vi "PH_ImageCalibrator.ProcState.vi"(0 "i ref in":refnum<vi>, 2 "state timeout":i32=-1, 4 "state":string, 5 "error in (no error)":errorcluster) -> (14 "i ref out":refnum<vi>, 18 "next state":string, 19 "error out":errorcluster)   [LabVIEW 2014, in "PH_ImageCalibrator.lvlib"]
doc: "This VI represents part of the internal state machine of the object. All methods that are needed to implement the required functionality of the state machine will be called from THIS VI. Add your code here."
uses:
  PH_ImageCalibrator.lvlib
  CSCore/CSSystem/CoreDefs/CoreDefs.error_type.ctl
  CSCore/CSSystem/CoreLib/CoreLib.lvlib
  CSCore/BaseSM/BaseSM.lvlib
  CSCore/BaseProcess/BaseProcess.lvlib
  <vilib>/vision/NI_Vision_Development_Module.lvlib
  CSCore/CSSystem/CSSystemLib/CSSystemLib.lvlib
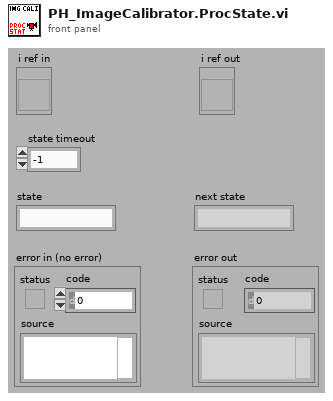
[diagram p1: front panel]
types:
  T1 = enum16{"simple", "synchronous", "asynchronous", "notification"}
  T2 = typedef "CoreDefs.error_type.ctl" = enum16{"no error", "can't load process", "can't unload process", "process does not exist", "can't install process", "can't remove process", "unknown function", "time out", "can't execute function", "duplicate queue name", "super not found", "caller queue invalid", "can't ping process", "unknown error", "VISA Error", "VISA timeout", "GPIB timeout", "GPIB error", "communication error", "data type mismatch", "can't read data from OPC server", "can't write data to OPC server", "OET error", "function not implemented", "process already exists", "invalid Shared Variable name", "error writing Shared Variable", "error reading Shared Variable", "invalid client name", "corrupt database", "unknown class", "call not authorized", "parameter out of range", "OET timeout: can't get data to modify", "invalid queue name", "requested operation incompatible with current state", "event undefined", "event disabled", "state undefined", "caller is not a friend", "EventBuilder: bad eventID", "EventBuilder: no DAQ devices", "a thread must not stop itself", "UNUSED ELEMENT4", "DiscArchiver: eventData incomplete", "DiscArchiver: eventData does not belong to run", "DiscArchiver: can't open file", "DiscArchiver: can't write to file", "DiscArchiver: available disc space low", "can't acquire semaphore", "error reading data from database", "notifier object is not existing", "can't register process", "can't unregister process", "illegal event type", "object disabled", "object already exists", "can't change state", "Instrument not found", "no connection to remote node", "invalid reference", "N/A", "UNUSED ELEMENT 1", "element not found", "illegal TCP/IP connection detected", "object does not exist", "invalid access ID", "unknown CS system", "invalid privilige", "unsupported data type", "unsupported server type", "IO server already exists", "Shared Variable already exists"}
  T3 = typedef "PH_ImageCalibrator.lvlib/PH_ImageCalibrator.i attribute.ctl" = cluster{"GUI Refs":cluster{"Available Cams":refnum<vi>, "OK":refnum<vi>, "Skip":refnum<vi>, "Repeat":refnum<vi>, "Cancel":refnum<vi>, "Length [mm]":refnum<vi>, "Energy [mJ]":refnum<vi>, "Dialog":refnum<vi>}, "Cam instances":string[], "Dark Pics":cluster{"#":i32, "BI taken":bool}, "Lin Cali":cluster{"Distance [Pixel]":dbl, "Distance [mm]":dbl, "Lin Cali Factor [mm/Pixel]":dbl}, "Energy Cali":cluster{"Pixelsum":dbl, "Energy [mJ]":dbl, "Energy Cali factor [mJ/Pixelsum]":dbl, "Underground subtracted?":bool, "#":i32}, "Images":cluster{"Background":T4, "Energy":T4}}
  T4 = typedef "IMAQ Image.ctl" = refnum<image>
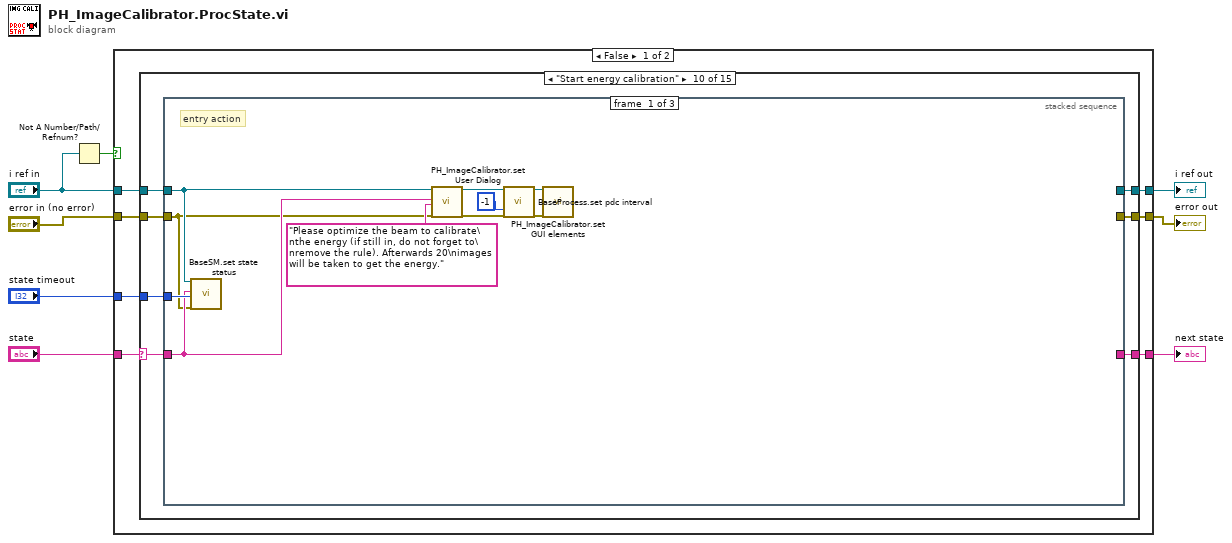
[diagram p0: block diagram]
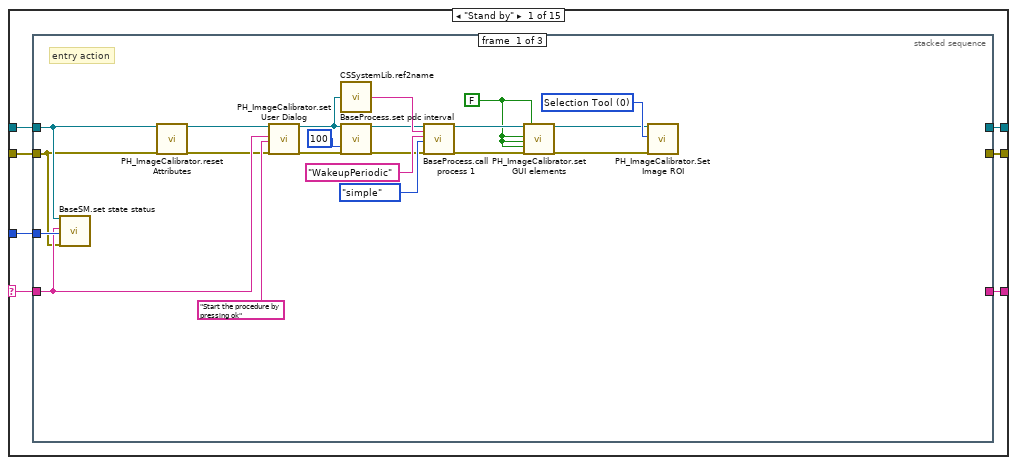
[diagram p2: hidden frame]
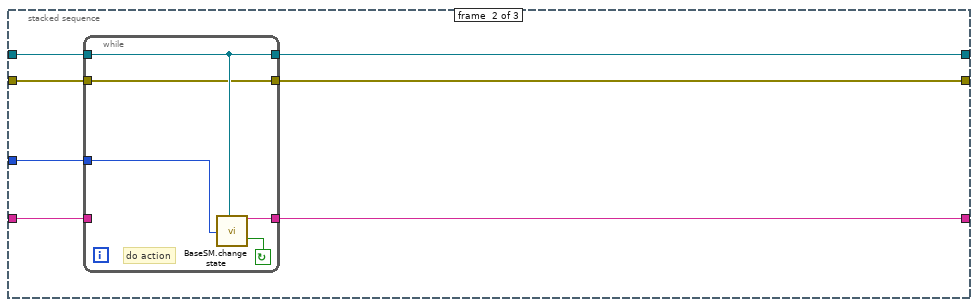
[diagram p3: hidden frame]
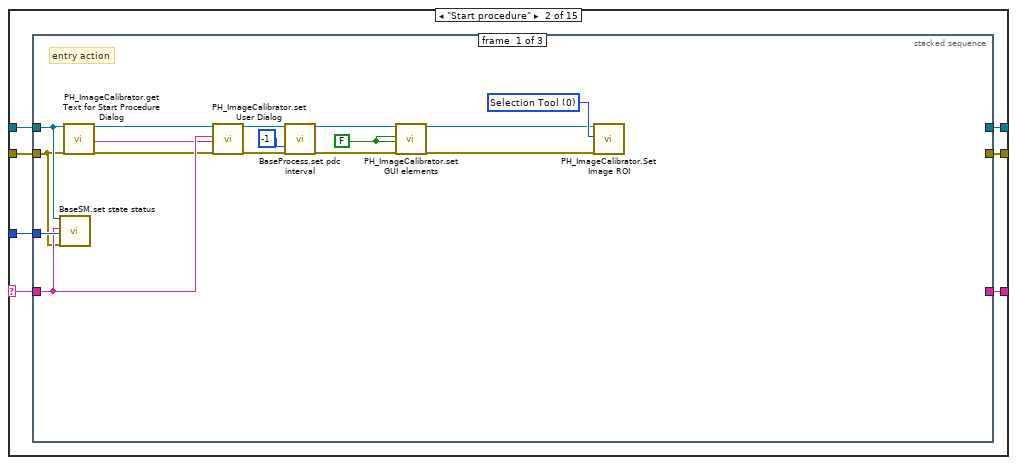
[diagram p5: hidden frame]
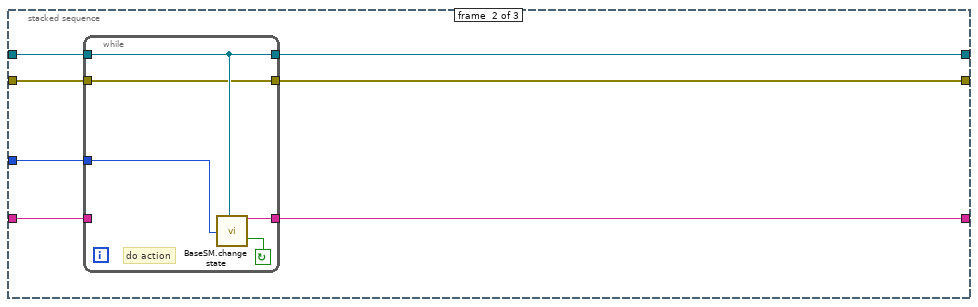
[diagram p6: hidden frame]
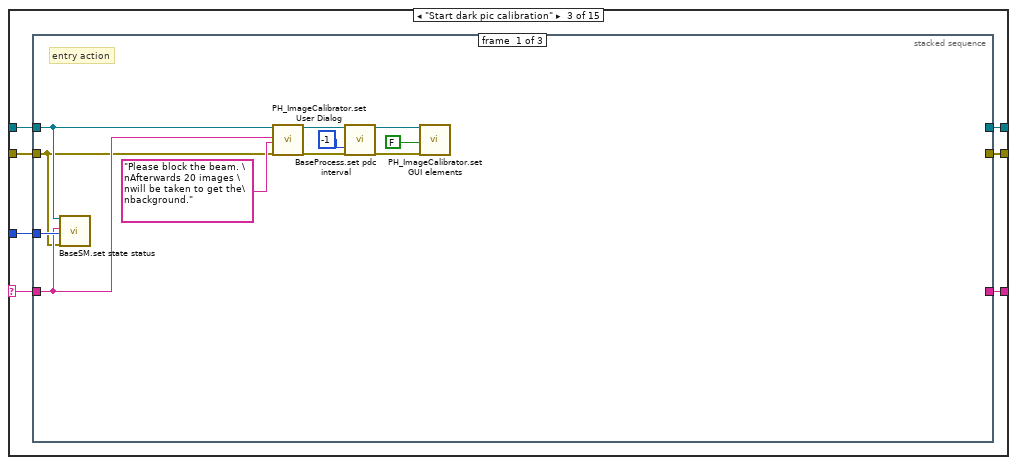
[diagram p8: hidden frame]
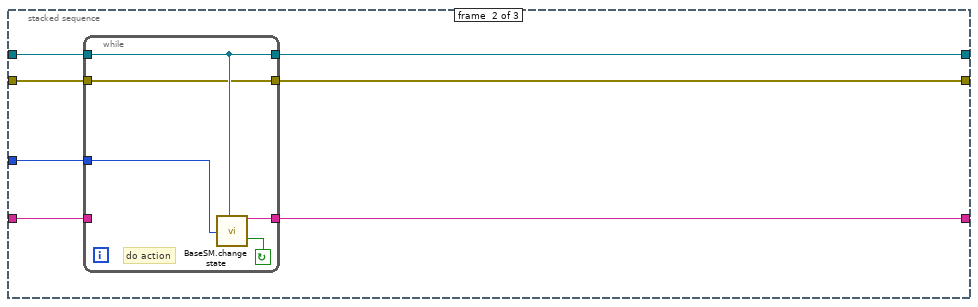
[diagram p9: hidden frame]
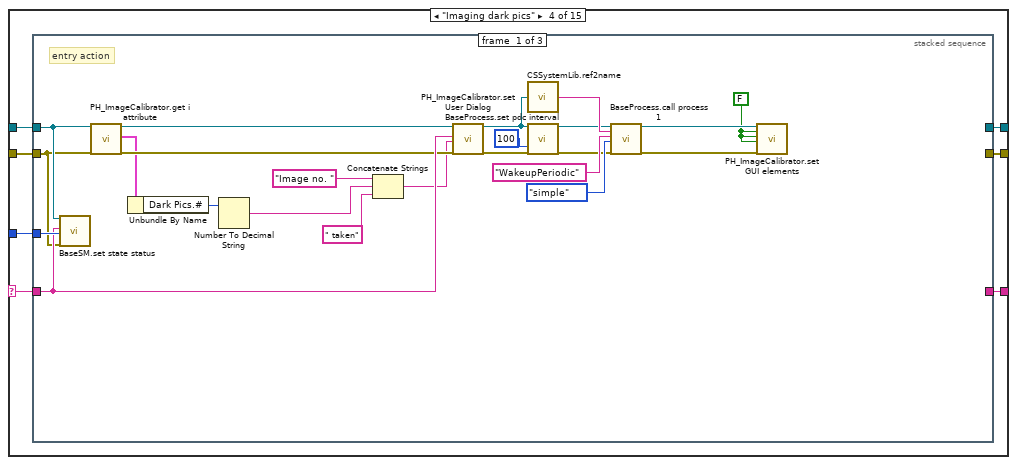
[diagram p11: hidden frame]
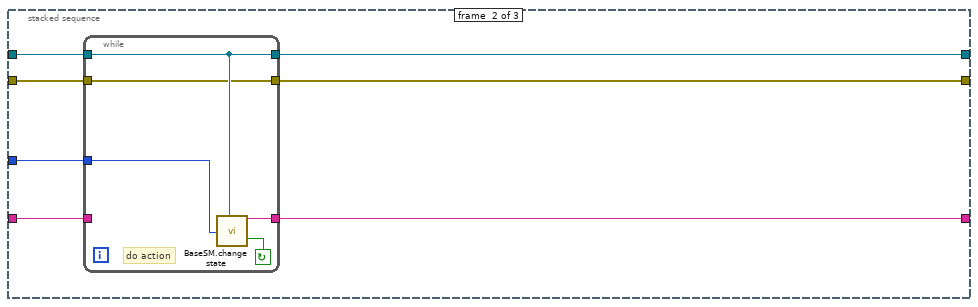
[diagram p12: hidden frame]
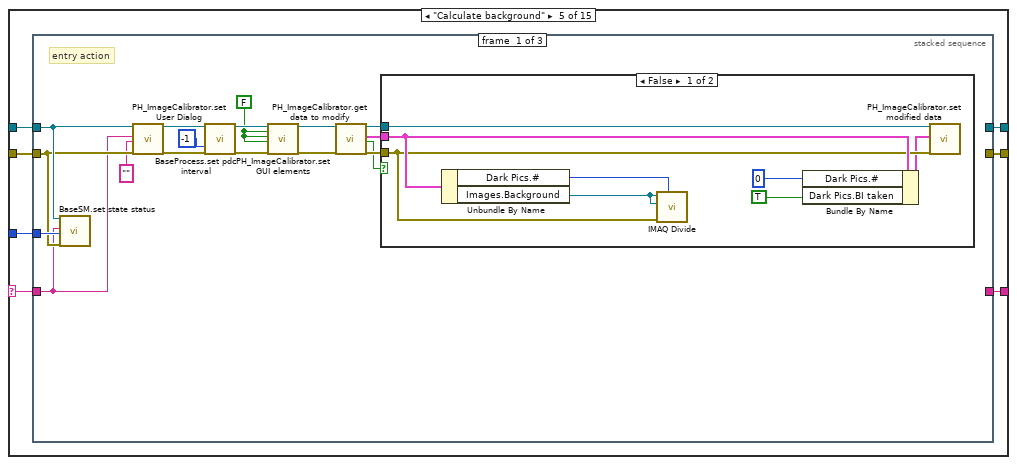
[diagram p14: hidden frame]
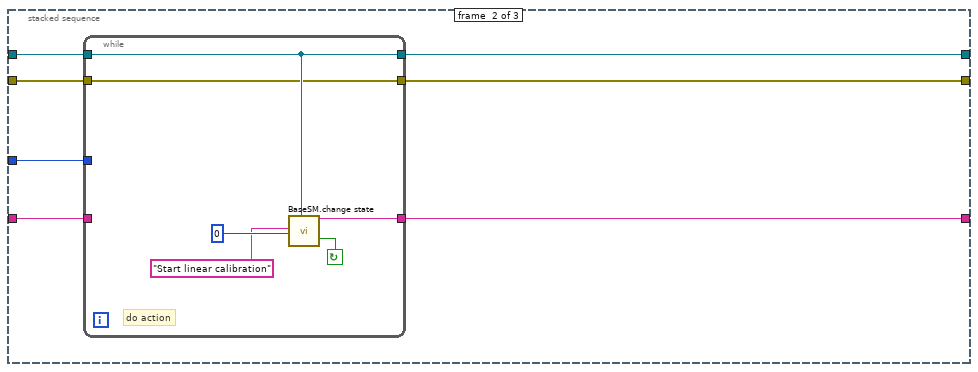
[diagram p16: hidden frame]
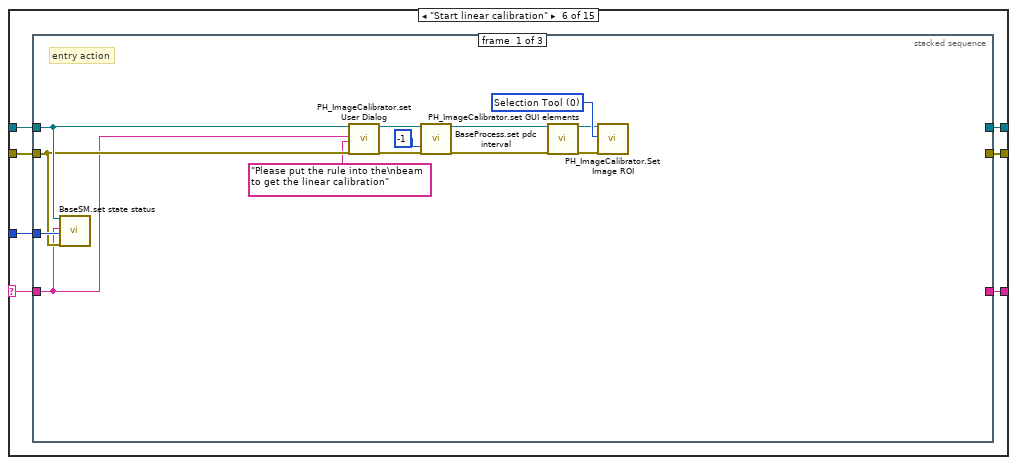
[diagram p18: hidden frame]
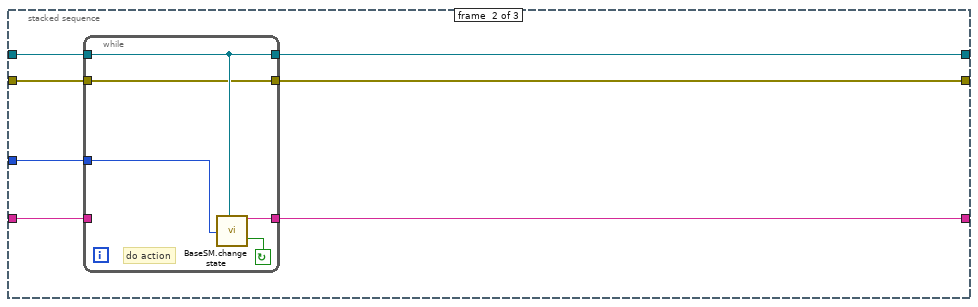
[diagram p19: hidden frame]
diagram:
  n1 = Not A Number/Path/Refnum?(number/path/refnum="i ref in") -> (NaN/Path/Refnum?=w2:bool)
  n2 = case shown="False" w2 {
    tunnel: "i ref in" -> [w15 w569]
    tunnel: [w14 w569] -> w8
    tunnel: "state" -> [w13 w566]
    tunnel: [w12 w566] -> w6
    tunnel: "state timeout" -> [w11 _]
    tunnel: "error in (no error)" -> [w10 _]
    tunnel: [w9 w567] -> w3
    frame False {
      n3 = case shown="\"Start energy calibration\"" w13 {
        selector: w13 -> [w22 w62 w97 w127 w169 w214 w246 w284 w316 w365 w394 w436 w484 w533 w560]
        tunnel: w15 -> [w20 w60 w95 w125 w167 w212 w244 w282 w314 w363 w392 w434 w482 w531 w565]
        tunnel: [w19 w59 w94 w124 w166 w211 w243 w281 w313 w362 w391 w433 w481 w530 w564] -> w14
        tunnel: [w21 w61 w96 w126 w168 w213 w245 w283 w315 w364 w393 w435 w483 w532 w559] -> w12
        tunnel: w11 -> [w18 w58 w93 w123 w165 w210 w242 w280 w312 w361 w390 w432 w480 w529 w561]
        tunnel: w10 -> [w17 w57 w92 w122 w164 w209 w241 w279 w311 w360 w389 w431 w479 w528 w563]
        tunnel: [w16 w56 w91 w121 w163 w208 w240 w278 w310 w359 w388 w430 w478 w527 w562] -> w9
        frame "Stand by" {
          n4 = stacked-sequence {
            tunnel: w22 -> [w42 w50 _]
            tunnel: [_ w49 _] -> w21
            tunnel: w20 -> [w29 w47 _]
            tunnel: [_ w46 _] -> w19
            tunnel: w18 -> [w43 w48 _]
            tunnel: w17 -> [w27 w44 _]
            tunnel: [_ w45 _] -> w16
            frame #0 {
              w25 = u32 0 items=["Zoom Tool"=8, "Selection Tool"=0, "Pan Tool"=9, "Point Tool"=1, "Line Tool"=2, "Rectangle Tool"=3, "Rotated Rectangle Tool"=12, "Polyline Tool"=10, "Polygon Tool"=5, "Freehand Tool"=11, "Closed Freehand Tool"=6, "Ellipse Tool"=4, "Annulus Tool"=7] ("ROI Tool")
              w30 = FALSE ("Cams disabled (true)")
              # "entry action"
              n5 = call "BaseSM.set state status.vi"("i ref in"=w29, "stateStatus"=w42, "ms timeout (10000)"=w43, "error in (no error)"=w27) -> ()  [unwired: 13 in, 3 out]
              n6 = call "PH_ImageCalibrator.reset Attributes.vi"("i ref in"=w29, "error in (no error)"=w27) -> ("i ref out"=w28:refnum<vi>, "error out"=w26:errorcluster)  [unwired: 16 in]
              n7 = call "PH_ImageCalibrator.set User Dialog.vi"("i ref in"=w28, "State"=w42, "Text"="Start the procedure by pressing ok", "error in (no error)"=w26) -> ("i ref out"=w34:refnum<vi>, "error out"=w36:errorcluster)  [unwired: 14 in]
              n8 = call "CSSystemLib.ref2name.vi"("obj refnum"=w34) -> ("name"=w40:string)
              n9 = call "BaseProcess.set pdc interval.vi"("i ref in"=w34, "PeriodicInterval [ms]"=100 ("PeriodicInterval"), "error in (no error)"=w36) -> ("i ref out"=w35:refnum<vi>, "error out"=w37:errorcluster)  [unwired: 14 in, 1 out]
              n10 = call "BaseProcess.call process 1.vi"("i ref in"=w35, "Object"=w40, "Selector"="WakeupPeriodic", "CallType"=T1."simple", "error in (no error)"=w37) -> ("i ref out"=w32:refnum<vi>, "error out"=w31:errorcluster)  [unwired: 12 in, 1 out]
              n11 = call "PH_ImageCalibrator.set GUI elements.vi"("i ref in"=w32, "skip visible (true)"=w30, "Repeat visible (true)"=w30, "Cancel visible (true)"=w30, "error in (no error)"=w31, "Cams disabled (true)"=w30) -> ("i ref out"=w24:refnum<vi>, "error out"=w23:errorcluster)  [unwired: 12 in]
              n12 = call "PH_ImageCalibrator.Set Image ROI.vi"("i ref in"=w24, "ROI Tool"=w25, "error in"=w23) -> ()  [unwired: 15 in, 2 out]
            }
            frame #1 {
              n13 = while {
                tunnel: w48 -> [w53]
                tunnel: [w55] -> w49
                tunnel: w50 -> [_]
                tunnel: w47 -> [w52]
                tunnel: [w52] -> w46
                tunnel: [w51] -> w45
                tunnel: w44 -> [w51]
                stop <- w54 continue-if-true
                # "do action"
                n14 = call "BaseSM.change state.vi"("wait time [ms]"=w53, "i ref in"=w52) -> ("next state"=w55:string, "continue loop"=w54:bool)  [unwired: 14 in, 2 out]
              }
            }
            frame #2 {
              # "exit action"
            }
          }
        }
        frame "Start procedure" {
          n15 = stacked-sequence {
            tunnel: w62 -> [w77 w85 _]
            tunnel: [_ w84 _] -> w61
            tunnel: w60 -> [w71 w82 _]
            tunnel: [_ w81 _] -> w59
            tunnel: w58 -> [w78 w83 _]
            tunnel: w57 -> [w69 w79 _]
            tunnel: [_ w80 _] -> w56
            frame #0 {
              w65 = u32 0 items=["Zoom Tool"=8, "Selection Tool"=0, "Pan Tool"=9, "Point Tool"=1, "Line Tool"=2, "Rectangle Tool"=3, "Rotated Rectangle Tool"=12, "Polyline Tool"=10, "Polygon Tool"=5, "Freehand Tool"=11, "Closed Freehand Tool"=6, "Ellipse Tool"=4, "Annulus Tool"=7] ("ROI Tool")
              w66 = FALSE ("Repeat visible (true)")
              # "entry action"
              n16 = call "BaseSM.set state status.vi"("i ref in"=w71, "stateStatus"=w77, "ms timeout (10000)"=w78, "error in (no error)"=w69) -> ()  [unwired: 13 in, 3 out]
              n17 = call "PH_ImageCalibrator.get Text for Start Procedure Dialog.vi"("i ref in"=w71, "error in (no error)"=w69) -> ("i ref out"=w70:refnum<vi>, "Dialog Start Procedure"=w67:string, "error out"=w68:errorcluster)  [unwired: 15 in]
              n18 = call "PH_ImageCalibrator.set User Dialog.vi"("i ref in"=w70, "State"=w77, "Text"=w67, "error in (no error)"=w68) -> ("i ref out"=w74:refnum<vi>, "error out"=w75:errorcluster)  [unwired: 14 in]
              n19 = call "BaseProcess.set pdc interval.vi"("i ref in"=w74, "PeriodicInterval [ms]"=-1 ("PeriodicInterval"), "error in (no error)"=w75) -> ("i ref out"=w73:refnum<vi>, "error out"=w72:errorcluster)  [unwired: 14 in, 1 out]
              n20 = call "PH_ImageCalibrator.set GUI elements.vi"("i ref in"=w73, "skip visible (true)"=w66, "Repeat visible (true)"=w66, "error in (no error)"=w72) -> ("i ref out"=w63:refnum<vi>, "error out"=w64:errorcluster)  [unwired: 14 in]
              n21 = call "PH_ImageCalibrator.Set Image ROI.vi"("i ref in"=w63, "ROI Tool"=w65, "error in"=w64) -> ()  [unwired: 15 in, 2 out]
            }
            frame #1 {
              n22 = while {
                tunnel: w83 -> [w88]
                tunnel: [w90] -> w84
                tunnel: w85 -> [_]
                tunnel: w82 -> [w87]
                tunnel: [w87] -> w81
                tunnel: [w86] -> w80
                tunnel: w79 -> [w86]
                stop <- w89 continue-if-true
                # "do action"
                n23 = call "BaseSM.change state.vi"("wait time [ms]"=w88, "i ref in"=w87) -> ("next state"=w90:string, "continue loop"=w89:bool)  [unwired: 14 in, 2 out]
              }
            }
            frame #2 {
              # "exit action"
            }
          }
        }
        frame "Start dark pic calibration" {
          n24 = stacked-sequence {
            tunnel: w97 -> [w107 w115 _]
            tunnel: [_ w114 _] -> w96
            tunnel: w95 -> [w99 w112 _]
            tunnel: [_ w111 _] -> w94
            tunnel: w93 -> [w108 w113 _]
            tunnel: w92 -> [w98 w109 _]
            tunnel: [_ w110 _] -> w91
            frame #0 {
              # "entry action"
              n25 = call "BaseSM.set state status.vi"("i ref in"=w99, "stateStatus"=w107, "ms timeout (10000)"=w108, "error in (no error)"=w98) -> ()  [unwired: 13 in, 3 out]
              n26 = call "PH_ImageCalibrator.set User Dialog.vi"("i ref in"=w99, "State"=w107, "Text"="Please block the beam. \nAfterwards 20 images \nwill be taken to get the\nbackground.", "error in (no error)"=w98) -> ("i ref out"=w104:refnum<vi>, "error out"=w105:errorcluster)  [unwired: 14 in]
              n27 = call "BaseProcess.set pdc interval.vi"("i ref in"=w104, "PeriodicInterval [ms]"=-1 ("PeriodicInterval"), "error in (no error)"=w105) -> ("i ref out"=w103:refnum<vi>, "error out"=w102:errorcluster)  [unwired: 14 in, 1 out]
              n28 = call "PH_ImageCalibrator.set GUI elements.vi"("i ref in"=w103, "Repeat visible (true)"=FALSE, "error in (no error)"=w102) -> ()  [unwired: 15 in, 2 out]
            }
            frame #1 {
              n29 = while {
                tunnel: w113 -> [w118]
                tunnel: [w120] -> w114
                tunnel: w115 -> [_]
                tunnel: w112 -> [w117]
                tunnel: [w117] -> w111
                tunnel: [w116] -> w110
                tunnel: w109 -> [w116]
                stop <- w119 continue-if-true
                # "do action"
                n30 = call "BaseSM.change state.vi"("wait time [ms]"=w118, "i ref in"=w117) -> ("next state"=w120:string, "continue loop"=w119:bool)  [unwired: 14 in, 2 out]
              }
            }
            frame #2 {
              # "exit action"
            }
          }
        }
        frame "Imaging dark pics" {
          n31 = stacked-sequence {
            tunnel: w127 -> [w149 w157 _]
            tunnel: [_ w156 _] -> w126
            tunnel: w125 -> [w148 w154 _]
            tunnel: [_ w153 _] -> w124
            tunnel: w123 -> [w150 w155 _]
            tunnel: w122 -> [w146 w151 _]
            tunnel: [_ w152 _] -> w121
            frame #0 {
              w128 = FALSE ("ok visible (true)")
              # "entry action"
              n32 = call "BaseSM.set state status.vi"("i ref in"=w148, "stateStatus"=w149, "ms timeout (10000)"=w150, "error in (no error)"=w146) -> ()  [unwired: 13 in, 3 out]
              n33 = call "PH_ImageCalibrator.get i attribute.vi"("i ref in"=w148, "error in (no error)"=w146) -> ("i ref out"=w147:refnum<vi>, "i attribute"=w144:T3, "error out"=w145:errorcluster)  [unwired: 15 in]
              n34 = Unbundle By Name(w144) -> ("Dark Pics.#"=w143:i32)
              n35 = Number To Decimal String(number=w143) -> (decimal integer string=w141:string)  [unwired: 1 in]
              n36 = Concatenate Strings("Image no. " ("string"), w141, " taken" ("string")) -> (w139:string)
              n37 = call "PH_ImageCalibrator.set User Dialog.vi"("i ref in"=w147, "State"=w149, "Text"=w139, "error in (no error)"=w145) -> ("i ref out"=w132:refnum<vi>, "error out"=w131:errorcluster)  [unwired: 14 in]
              n38 = call "CSSystemLib.ref2name.vi"("obj refnum"=w132) -> ("name"=w137:string)
              n39 = call "BaseProcess.set pdc interval.vi"("i ref in"=w132, "PeriodicInterval [ms]"=100 ("PeriodicInterval"), "error in (no error)"=w131) -> ("i ref out"=w133:refnum<vi>, "error out"=w134:errorcluster)  [unwired: 14 in, 1 out]
              n40 = call "BaseProcess.call process 1.vi"("i ref in"=w133, "Object"=w137, "Selector"="WakeupPeriodic", "CallType"=T1."simple", "error in (no error)"=w134) -> ("i ref out"=w130:refnum<vi>, "error out"=w129:errorcluster)  [unwired: 12 in, 1 out]
              n41 = call "PH_ImageCalibrator.set GUI elements.vi"("i ref in"=w130, "ok visible (true)"=w128, "skip visible (true)"=w128, "Repeat visible (true)"=w128, "error in (no error)"=w129) -> ()  [unwired: 13 in, 2 out]
            }
            frame #1 {
              n42 = while {
                tunnel: w155 -> [w160]
                tunnel: [w162] -> w156
                tunnel: w157 -> [_]
                tunnel: w154 -> [w159]
                tunnel: [w159] -> w153
                tunnel: [w158] -> w152
                tunnel: w151 -> [w158]
                stop <- w161 continue-if-true
                # "do action"
                n43 = call "BaseSM.change state.vi"("wait time [ms]"=w160, "i ref in"=w159) -> ("next state"=w162:string, "continue loop"=w161:bool)  [unwired: 14 in, 2 out]
              }
            }
            frame #2 {
              # "exit action"
            }
          }
        }
        frame "Calculate background" {
          n44 = stacked-sequence {
            tunnel: w169 -> [w183 w201 _]
            tunnel: [_ w200 _] -> w168
            tunnel: w167 -> [w185 w198 _]
            tunnel: [_ w197 _] -> w166
            tunnel: w165 -> [w186 w199 _]
            tunnel: w164 -> [w184 w195 _]
            tunnel: [_ w196 _] -> w163
            frame #0 {
              w176 = FALSE ("ok visible (true)")
              # "entry action"
              n45 = call "BaseSM.set state status.vi"("i ref in"=w185, "stateStatus"=w183, "ms timeout (10000)"=w186, "error in (no error)"=w184) -> ()  [unwired: 13 in, 3 out]
              n46 = call "PH_ImageCalibrator.set User Dialog.vi"("i ref in"=w185, "State"=w183, "Text"="", "error in (no error)"=w184) -> ("i ref out"=w180:refnum<vi>, "error out"=w181:errorcluster)  [unwired: 14 in]
              n47 = call "BaseProcess.set pdc interval.vi"("i ref in"=w180, "PeriodicInterval [ms]"=-1 ("PeriodicInterval"), "error in (no error)"=w181) -> ("i ref out"=w179:refnum<vi>, "error out"=w178:errorcluster)  [unwired: 14 in, 1 out]
              n48 = call "PH_ImageCalibrator.set GUI elements.vi"("i ref in"=w179, "ok visible (true)"=w176, "skip visible (true)"=w176, "Repeat visible (true)"=w176, "error in (no error)"=w178) -> ("i ref out"=w175:refnum<vi>, "error out"=w174:errorcluster)  [unwired: 13 in]
              n49 = call "PH_ImageCalibrator.get data to modify.vi"("i ref in"=w175, "error in (no error)"=w174) -> ("i ref out"=w170:refnum<vi>, "i attribute"=w173:T3, "timed out"=w171:bool, "error out"=w172:errorcluster)  [unwired: 14 in]
              n50 = case shown="False" w171 {
                tunnel: w173 -> [w193 _]
                tunnel: w172 -> [w191 _]
                tunnel: w170 -> [w192 _]
                frame False {
                  n51 = Unbundle By Name(w193) -> ("Dark Pics.#"=w194:i32, "Images.Background"=w187:T4)
                  n52 = call "IMAQ Divide"("Image Src A"=w187, "Constant"=w194, "Image Dst"=w187, "error in (no error)"=w191) -> ()  [unwired: 3 in, 2 out]
                  n53 = Bundle By Name(cluster=w193, "Dark Pics.#"=0, "Dark Pics.BI taken"=TRUE) -> (w190:T3)
                  n54 = call "PH_ImageCalibrator.set modified data.vi"("i ref in"=w192, "i attribute"=w190, "error in (no error)"=w191) -> ()  [unwired: 15 in, 2 out]
                }
                frame True {
                }
              }
            }
            frame #1 {
              n55 = while {
                tunnel: w199 -> [_]
                tunnel: [w207] -> w200
                tunnel: w201 -> [_]
                tunnel: w198 -> [w205]
                tunnel: [w205] -> w197
                tunnel: [w204] -> w196
                tunnel: w195 -> [w204]
                stop <- w206 continue-if-true
                # "do action"
                n56 = call "BaseSM.change state.vi"("default state"="Start linear calibration", "wait time [ms]"=0 ("wait time"), "i ref in"=w205) -> ("next state"=w207:string, "continue loop"=w206:bool)  [unwired: 13 in, 2 out]
              }
            }
            frame #2 {
              # "exit action"
            }
          }
        }
        frame "Start linear calibration" {
          n57 = stacked-sequence {
            tunnel: w214 -> [w224 w234 _]
            tunnel: [_ w233 _] -> w213
            tunnel: w212 -> [w226 w231 _]
            tunnel: [_ w230 _] -> w211
            tunnel: w210 -> [w227 w232 _]
            tunnel: w209 -> [w225 w228 _]
            tunnel: [_ w229 _] -> w208
            frame #0 {
              w217 = u32 0 items=["Zoom Tool"=8, "Selection Tool"=0, "Pan Tool"=9, "Point Tool"=1, "Line Tool"=2, "Rectangle Tool"=3, "Rotated Rectangle Tool"=12, "Polyline Tool"=10, "Polygon Tool"=5, "Freehand Tool"=11, "Closed Freehand Tool"=6, "Ellipse Tool"=4, "Annulus Tool"=7] ("ROI Tool")
              # "entry action"
              n58 = call "BaseSM.set state status.vi"("i ref in"=w226, "stateStatus"=w224, "ms timeout (10000)"=w227, "error in (no error)"=w225) -> ()  [unwired: 13 in, 3 out]
              n59 = call "PH_ImageCalibrator.set User Dialog.vi"("i ref in"=w226, "State"=w224, "Text"="Please put the rule into the\nbeam to get the linear calibration", "error in (no error)"=w225) -> ("i ref out"=w221:refnum<vi>, "error out"=w222:errorcluster)  [unwired: 14 in]
              n60 = call "BaseProcess.set pdc interval.vi"("i ref in"=w221, "PeriodicInterval [ms]"=-1 ("PeriodicInterval"), "error in (no error)"=w222) -> ("i ref out"=w220:refnum<vi>, "error out"=w219:errorcluster)  [unwired: 14 in, 1 out]
              n61 = call "PH_ImageCalibrator.set GUI elements.vi"("i ref in"=w220, "error in (no error)"=w219) -> ("i ref out"=w215:refnum<vi>, "error out"=w216:errorcluster)  [unwired: 16 in]
              n62 = call "PH_ImageCalibrator.Set Image ROI.vi"("i ref in"=w215, "ROI Tool"=w217, "error in"=w216) -> ()  [unwired: 15 in, 2 out]
            }
            frame #1 {
              n63 = while {
                tunnel: w232 -> [w237]
                tunnel: [w239] -> w233
                tunnel: w234 -> [_]
                tunnel: w231 -> [w236]
                tunnel: [w236] -> w230
                tunnel: [w235] -> w229
                tunnel: w228 -> [w235]
                stop <- w238 continue-if-true
                # "do action"
                n64 = call "BaseSM.change state.vi"("wait time [ms]"=w237, "i ref in"=w236) -> ("next state"=w239:string, "continue loop"=w238:bool)  [unwired: 14 in, 2 out]
              }
            }
            frame #2 {
              # "exit action"
            }
          }
        }
        frame "Imaging rule" {
          n65 = stacked-sequence {
            tunnel: w246 -> [w262 w272 _]
            tunnel: [_ w271 _] -> w245
            tunnel: w244 -> [w264 w269 _]
            tunnel: [_ w268 _] -> w243
            tunnel: w242 -> [w265 w270 _]
            tunnel: w241 -> [w263 w266 _]
            tunnel: [_ w267 _] -> w240
            frame #0 {
              w250 = u32 2 items=["Zoom Tool"=8, "Selection Tool"=0, "Pan Tool"=9, "Point Tool"=1, "Line Tool"=2, "Rectangle Tool"=3, "Rotated Rectangle Tool"=12, "Polyline Tool"=10, "Polygon Tool"=5, "Freehand Tool"=11, "Closed Freehand Tool"=6, "Ellipse Tool"=4, "Annulus Tool"=7] ("ROI Tool")
              # "entry action"
              n66 = call "BaseSM.set state status.vi"("i ref in"=w264, "stateStatus"=w262, "ms timeout (10000)"=w265, "error in (no error)"=w263) -> ()  [unwired: 13 in, 3 out]
              n67 = call "PH_ImageCalibrator.set User Dialog.vi"("i ref in"=w264, "State"=w262, "Text"="Please set a line as rule", "error in (no error)"=w263) -> ("i ref out"=w255:refnum<vi>, "error out"=w254:errorcluster)  [unwired: 14 in]
              n68 = call "CSSystemLib.ref2name.vi"("obj refnum"=w255) -> ("name"=w260:string)
              n69 = call "BaseProcess.set pdc interval.vi"("i ref in"=w255, "PeriodicInterval [ms]"=100 ("PeriodicInterval"), "error in (no error)"=w254) -> ("i ref out"=w256:refnum<vi>, "error out"=w257:errorcluster)  [unwired: 14 in, 1 out]
              n70 = call "BaseProcess.call process 1.vi"("i ref in"=w256, "Object"=w260, "Selector"="WakeupPeriodic", "CallType"=T1."simple", "error in (no error)"=w257) -> ("i ref out"=w253:refnum<vi>, "error out"=w252:errorcluster)  [unwired: 12 in, 1 out]
              n71 = call "PH_ImageCalibrator.set GUI elements.vi"("i ref in"=w253, "Repeat visible (true)"=FALSE, "error in (no error)"=w252) -> ("i ref out"=w248:refnum<vi>, "error out"=w249:errorcluster)  [unwired: 15 in]
              n72 = call "PH_ImageCalibrator.Set Image ROI.vi"("i ref in"=w248, "ROI Tool"=w250, "error in"=w249) -> ()  [unwired: 15 in, 2 out]
            }
            frame #1 {
              n73 = while {
                tunnel: w270 -> [w275]
                tunnel: [w277] -> w271
                tunnel: w272 -> [_]
                tunnel: w269 -> [w274]
                tunnel: [w274] -> w268
                tunnel: [w273] -> w267
                tunnel: w266 -> [w273]
                stop <- w276 continue-if-true
                # "do action"
                n74 = call "BaseSM.change state.vi"("wait time [ms]"=w275, "i ref in"=w274) -> ("next state"=w277:string, "continue loop"=w276:bool)  [unwired: 14 in, 2 out]
              }
            }
            frame #2 {
              # "exit action"
            }
          }
        }
        frame "Enter distance" {
          n75 = stacked-sequence {
            tunnel: w284 -> [w296 w304 _]
            tunnel: [_ w303 _] -> w283
            tunnel: w282 -> [w287 w301 _]
            tunnel: [_ w300 _] -> w281
            tunnel: w280 -> [w297 w302 _]
            tunnel: w279 -> [w288 w298 _]
            tunnel: [_ w299 _] -> w278
            frame #0 {
              w289 = FALSE ("Length not visible (true)")
              # "entry action"
              n76 = call "BaseSM.set state status.vi"("i ref in"=w287, "stateStatus"=w296, "ms timeout (10000)"=w297, "error in (no error)"=w288) -> ()  [unwired: 13 in, 3 out]
              n77 = call "PH_ImageCalibrator.set Distance in Pixel.vi"("i ref in"=w287, "error in (no error)"=w288) -> ("i ref out"=w286:refnum<vi>, "error out"=w285:errorcluster)  [unwired: 16 in]
              n78 = call "PH_ImageCalibrator.set User Dialog.vi"("i ref in"=w286, "State"=w296, "Text"="Please enter the length (in mm) for a nearfield cam,\nor the angle (in mrad) in case of a farfield cam,\nmarked within the auxiliary window", "error in (no error)"=w285) -> ("i ref out"=w293:refnum<vi>, "error out"=w294:errorcluster)  [unwired: 14 in]
              n79 = call "BaseProcess.set pdc interval.vi"("i ref in"=w293, "PeriodicInterval [ms]"=-1 ("PeriodicInterval"), "error in (no error)"=w294) -> ("i ref out"=w292:refnum<vi>, "error out"=w291:errorcluster)  [unwired: 14 in, 1 out]
              n80 = call "PH_ImageCalibrator.set GUI elements.vi"("i ref in"=w292, "ok visible (true)"=w289, "error in (no error)"=w291, "Length not visible (true)"=w289) -> ()  [unwired: 14 in, 2 out]
            }
            frame #1 {
              n81 = while {
                tunnel: w302 -> [w307]
                tunnel: [w309] -> w303
                tunnel: w304 -> [_]
                tunnel: w301 -> [w306]
                tunnel: [w306] -> w300
                tunnel: [w305] -> w299
                tunnel: w298 -> [w305]
                stop <- w308 continue-if-true
                # "do action"
                n82 = call "BaseSM.change state.vi"("wait time [ms]"=w307, "i ref in"=w306) -> ("next state"=w309:string, "continue loop"=w308:bool)  [unwired: 14 in, 2 out]
              }
            }
            frame #2 {
              # "exit action"
            }
          }
        }
        frame "Calculate linear calibration" {
          n83 = stacked-sequence {
            tunnel: w316 -> [w330 w352 _]
            tunnel: [_ w351 _] -> w315
            tunnel: w314 -> [w332 w349 _]
            tunnel: [_ w348 _] -> w313
            tunnel: w312 -> [w333 w350 _]
            tunnel: w311 -> [w331 w346 _]
            tunnel: [_ w347 _] -> w310
            frame #0 {
              w323 = FALSE ("ok visible (true)")
              # "entry action"
              n84 = call "BaseSM.set state status.vi"("i ref in"=w332, "stateStatus"=w330, "ms timeout (10000)"=w333, "error in (no error)"=w331) -> ()  [unwired: 13 in, 3 out]
              n85 = call "PH_ImageCalibrator.set User Dialog.vi"("i ref in"=w332, "State"=w330, "Text"="", "error in (no error)"=w331) -> ("i ref out"=w327:refnum<vi>, "error out"=w328:errorcluster)  [unwired: 14 in]
              n86 = call "BaseProcess.set pdc interval.vi"("i ref in"=w327, "PeriodicInterval [ms]"=-1 ("PeriodicInterval"), "error in (no error)"=w328) -> ("i ref out"=w326:refnum<vi>, "error out"=w325:errorcluster)  [unwired: 14 in, 1 out]
              n87 = call "PH_ImageCalibrator.set GUI elements.vi"("i ref in"=w326, "ok visible (true)"=w323, "skip visible (true)"=w323, "Repeat visible (true)"=w323, "error in (no error)"=w325) -> ("i ref out"=w318:refnum<vi>, "error out"=w317:errorcluster)  [unwired: 13 in]
              n88 = call "PH_ImageCalibrator.get data to modify.vi"("i ref in"=w318, "error in (no error)"=w317) -> ("i ref out"=w322:refnum<vi>, "i attribute"=w319:T3, "timed out"=w320:bool, "error out"=w321:errorcluster)  [unwired: 14 in]
              n89 = case shown="False" w320 {
                tunnel: w322 -> [w341 _]
                tunnel: w321 -> [w340 _]
                tunnel: w319 -> [w338 _]
                frame False {
                  n90 = Unbundle By Name(w338) -> ("Lin Cali.Distance [mm]"=w337:dbl, "Lin Cali.Distance [Pixel]"=w335:dbl)
                  n91 = Not Equal To 0?(x=w335) -> (x != 0?=w334:bool)
                  n92 = case shown="False" w334 {
                    tunnel: w337 -> [_ w345]
                    tunnel: w335 -> [_ w344]
                    tunnel: [1.0 w343] -> w336
                    frame False {
                    }
                    frame True {
                      n93 = Divide(x=w345, y=w344) -> (x/y=w343:dbl)
                    }
                  }
                  n94 = Bundle By Name(cluster=w338, "Lin Cali.Lin Cali Factor [mm/Pixel]"=w336) -> (w339:T3)
                  n95 = call "PH_ImageCalibrator.set modified data.vi"("i ref in"=w341, "i attribute"=w339, "error in (no error)"=w340) -> ()  [unwired: 15 in, 2 out]
                }
                frame True {
                }
              }
            }
            frame #1 {
              n96 = while {
                tunnel: w350 -> [_]
                tunnel: [w358] -> w351
                tunnel: w352 -> [_]
                tunnel: w349 -> [w356]
                tunnel: [w356] -> w348
                tunnel: [w355] -> w347
                tunnel: w346 -> [w355]
                stop <- w357 continue-if-true
                # "do action"
                n97 = call "BaseSM.change state.vi"("default state"="Start energy calibration", "wait time [ms]"=0 ("wait time"), "i ref in"=w356) -> ("next state"=w358:string, "continue loop"=w357:bool)  [unwired: 13 in, 2 out]
              }
            }
            frame #2 {
              # "exit action"
            }
          }
        }
        frame "Start energy calibration" {
          n98 = stacked-sequence {
            tunnel: w365 -> [w374 w382 _]
            tunnel: [_ w381 _] -> w364
            tunnel: w363 -> [w367 w379 _]
            tunnel: [_ w378 _] -> w362
            tunnel: w361 -> [w375 w380 _]
            tunnel: w360 -> [w366 w376 _]
            tunnel: [_ w377 _] -> w359
            frame #0 {
              # "entry action"
              n99 = call "BaseSM.set state status.vi"("i ref in"=w367, "stateStatus"=w374, "ms timeout (10000)"=w375, "error in (no error)"=w366) -> ()  [unwired: 13 in, 3 out]
              n100 = call "PH_ImageCalibrator.set User Dialog.vi"("i ref in"=w367, "State"=w374, "Text"="Please optimize the beam to calibrate\nthe energy (if still in, do not forget to\nremove the rule). Afterwards 20\nimages will be taken to get the energy.", "error in (no error)"=w366) -> ("i ref out"=w371:refnum<vi>, "error out"=w372:errorcluster)  [unwired: 14 in]
              n101 = call "BaseProcess.set pdc interval.vi"("i ref in"=w371, "PeriodicInterval [ms]"=-1 ("PeriodicInterval"), "error in (no error)"=w372) -> ("i ref out"=w370:refnum<vi>, "error out"=w369:errorcluster)  [unwired: 14 in, 1 out]
              n102 = call "PH_ImageCalibrator.set GUI elements.vi"("i ref in"=w370, "error in (no error)"=w369) -> ()  [unwired: 16 in, 2 out]
            }
            frame #1 {
              n103 = while {
                tunnel: w380 -> [w383]
                tunnel: [w387] -> w381
                tunnel: w382 -> [_]
                tunnel: w379 -> [w385]
                tunnel: [w385] -> w378
                tunnel: [w384] -> w377
                tunnel: w376 -> [w384]
                stop <- w386 continue-if-true
                # "do action"
                n104 = call "BaseSM.change state.vi"("wait time [ms]"=w383, "i ref in"=w385) -> ("next state"=w387:string, "continue loop"=w386:bool)  [unwired: 14 in, 2 out]
              }
            }
            frame #2 {
              # "exit action"
            }
          }
        }
        frame "Imaging beam" {
          n105 = stacked-sequence {
            tunnel: w394 -> [w416 w424 _]
            tunnel: [_ w423 _] -> w393
            tunnel: w392 -> [w399 w421 _]
            tunnel: [_ w420 _] -> w391
            tunnel: w390 -> [w417 w422 _]
            tunnel: w389 -> [w397 w418 _]
            tunnel: [_ w419 _] -> w388
            frame #0 {
              w405 = FALSE ("ok visible (true)")
              # "entry action"
              n106 = call "BaseSM.set state status.vi"("i ref in"=w399, "stateStatus"=w416, "ms timeout (10000)"=w417, "error in (no error)"=w397) -> ()  [unwired: 13 in, 3 out]
              n107 = call "PH_ImageCalibrator.get i attribute.vi"("i ref in"=w399, "error in (no error)"=w397) -> ("i ref out"=w398:refnum<vi>, "i attribute"=w404:T3, "error out"=w396:errorcluster)  [unwired: 15 in]
              n108 = Unbundle By Name(w404) -> ("Energy Cali.#"=w403:i32)
              n109 = Number To Decimal String(number=w403) -> (decimal integer string=w401:string)  [unwired: 1 in]
              n110 = Concatenate Strings("Image no. " ("string"), w401, " taken" ("string")) -> (w395:string)
              n111 = call "PH_ImageCalibrator.set User Dialog.vi"("i ref in"=w398, "State"=w416, "Text"=w395, "error in (no error)"=w396) -> ("i ref out"=w409:refnum<vi>, "error out"=w408:errorcluster)  [unwired: 14 in]
              n112 = call "CSSystemLib.ref2name.vi"("obj refnum"=w409) -> ("name"=w414:string)
              n113 = call "BaseProcess.set pdc interval.vi"("i ref in"=w409, "PeriodicInterval [ms]"=100 ("PeriodicInterval"), "error in (no error)"=w408) -> ("i ref out"=w410:refnum<vi>, "error out"=w411:errorcluster)  [unwired: 14 in, 1 out]
              n114 = call "BaseProcess.call process 1.vi"("i ref in"=w410, "Object"=w414, "Selector"="WakeupPeriodic", "CallType"=T1."simple", "error in (no error)"=w411) -> ("i ref out"=w406:refnum<vi>, "error out"=w407:errorcluster)  [unwired: 12 in, 1 out]
              n115 = call "PH_ImageCalibrator.set GUI elements.vi"("i ref in"=w406, "ok visible (true)"=w405, "skip visible (true)"=w405, "Repeat visible (true)"=w405, "error in (no error)"=w407) -> ()  [unwired: 13 in, 2 out]
            }
            frame #1 {
              n116 = while {
                tunnel: w422 -> [w427]
                tunnel: [w429] -> w423
                tunnel: w424 -> [_]
                tunnel: w421 -> [w426]
                tunnel: [w426] -> w420
                tunnel: [w425] -> w419
                tunnel: w418 -> [w425]
                stop <- w428 continue-if-true
                # "do action"
                n117 = call "BaseSM.change state.vi"("wait time [ms]"=w427, "i ref in"=w426) -> ("next state"=w429:string, "continue loop"=w428:bool)  [unwired: 14 in, 2 out]
              }
            }
            frame #2 {
              # "exit action"
            }
          }
        }
        frame "Enter energy" {
          n118 = stacked-sequence {
            tunnel: w436 -> [w452 w472 _]
            tunnel: [_ w471 _] -> w435
            tunnel: w434 -> [w440 w469 _]
            tunnel: [_ w468 _] -> w433
            tunnel: w432 -> [w453 w470 _]
            tunnel: w431 -> [w438 w466 _]
            tunnel: [_ w467 _] -> w430
            frame #0 {
              w445 = FALSE ("Energy not visible (true)")
              # "entry action"
              n119 = call "BaseSM.set state status.vi"("i ref in"=w440, "stateStatus"=w452, "ms timeout (10000)"=w453, "error in (no error)"=w438) -> ()  [unwired: 13 in, 3 out]
              n120 = call "PH_ImageCalibrator.get data to modify.vi"("i ref in"=w440, "error in (no error)"=w438) -> ("i ref out"=w441:refnum<vi>, "i attribute"=w444:T3, "timed out"=w442:bool, "error out"=w443:errorcluster)  [unwired: 14 in]
              n121 = case shown="False" w442 {
                tunnel: w444 -> [w463 _]
                tunnel: w443 -> [w461 w464]
                tunnel: w441 -> [w462 w465]
                tunnel: [w455 w465] -> w439
                tunnel: [w454 w464] -> w437
                frame False {
                  n122 = Unbundle By Name(w463) -> ("Energy Cali.Pixelsum"=w458:dbl, "Energy Cali.#"=w457:i32)
                  n123 = Divide(x=w458, y=w457) -> (x/y=w456:dbl)
                  n124 = Bundle By Name(cluster=w463, "Energy Cali.#"=0 ("Dark Pics.#"), "Energy Cali.Pixelsum"=w456) -> (w460:T3)
                  n125 = call "PH_ImageCalibrator.set modified data.vi"("i ref in"=w462, "i attribute"=w460, "error in (no error)"=w461) -> ("i ref out"=w455:refnum<vi>, "error out"=w454:errorcluster)  [unwired: 15 in]
                }
                frame True {
                }
              }
              n126 = call "PH_ImageCalibrator.set User Dialog.vi"("i ref in"=w439, "State"=w452, "Text"="Please enter the energy (in mJ)\ncorresponding to the image.", "error in (no error)"=w437) -> ("i ref out"=w449:refnum<vi>, "error out"=w450:errorcluster)  [unwired: 14 in]
              n127 = call "BaseProcess.set pdc interval.vi"("i ref in"=w449, "PeriodicInterval [ms]"=-1 ("PeriodicInterval"), "error in (no error)"=w450) -> ("i ref out"=w448:refnum<vi>, "error out"=w447:errorcluster)  [unwired: 14 in, 1 out]
              n128 = call "PH_ImageCalibrator.set GUI elements.vi"("i ref in"=w448, "ok visible (true)"=w445, "error in (no error)"=w447, "Energy not visible (true)"=w445) -> ()  [unwired: 14 in, 2 out]
            }
            frame #1 {
              n129 = while {
                tunnel: w470 -> [w475]
                tunnel: [w477] -> w471
                tunnel: w472 -> [_]
                tunnel: w469 -> [w474]
                tunnel: [w474] -> w468
                tunnel: [w473] -> w467
                tunnel: w466 -> [w473]
                stop <- w476 continue-if-true
                # "do action"
                n130 = call "BaseSM.change state.vi"("wait time [ms]"=w475, "i ref in"=w474) -> ("next state"=w477:string, "continue loop"=w476:bool)  [unwired: 14 in, 2 out]
              }
            }
            frame #2 {
              # "exit action"
            }
          }
        }
        frame "Calculate energy" {
          n131 = stacked-sequence {
            tunnel: w484 -> [w498 w520 _]
            tunnel: [_ w519 _] -> w483
            tunnel: w482 -> [w500 w517 _]
            tunnel: [_ w516 _] -> w481
            tunnel: w480 -> [w501 w518 _]
            tunnel: w479 -> [w499 w514 _]
            tunnel: [_ w515 _] -> w478
            frame #0 {
              w491 = FALSE ("ok visible (true)")
              # "entry action"
              n132 = call "BaseSM.set state status.vi"("i ref in"=w500, "stateStatus"=w498, "ms timeout (10000)"=w501, "error in (no error)"=w499) -> ()  [unwired: 13 in, 3 out]
              n133 = call "PH_ImageCalibrator.set User Dialog.vi"("i ref in"=w500, "State"=w498, "Text"="", "error in (no error)"=w499) -> ("i ref out"=w495:refnum<vi>, "error out"=w496:errorcluster)  [unwired: 14 in]
              n134 = call "BaseProcess.set pdc interval.vi"("i ref in"=w495, "PeriodicInterval [ms]"=-1 ("PeriodicInterval"), "error in (no error)"=w496) -> ("i ref out"=w494:refnum<vi>, "error out"=w493:errorcluster)  [unwired: 14 in, 1 out]
              n135 = call "PH_ImageCalibrator.set GUI elements.vi"("i ref in"=w494, "ok visible (true)"=w491, "skip visible (true)"=w491, "Repeat visible (true)"=w491, "error in (no error)"=w493) -> ("i ref out"=w486:refnum<vi>, "error out"=w485:errorcluster)  [unwired: 13 in]
              n136 = call "PH_ImageCalibrator.get data to modify.vi"("i ref in"=w486, "error in (no error)"=w485) -> ("i ref out"=w490:refnum<vi>, "i attribute"=w487:T3, "timed out"=w488:bool, "error out"=w489:errorcluster)  [unwired: 14 in]
              n137 = case shown="False" w488 {
                tunnel: w490 -> [w509 _]
                tunnel: w489 -> [w508 _]
                tunnel: w487 -> [w506 _]
                frame False {
                  n138 = Unbundle By Name(w506) -> ("Energy Cali.Energy [mJ]"=w505:dbl, "Energy Cali.Pixelsum"=w503:dbl)
                  n139 = Not Equal To 0?(x=w503) -> (x != 0?=w502:bool)
                  n140 = case shown="True" w502 {
                    tunnel: w505 -> [_ w513]
                    tunnel: [1.0 w512] -> w504
                    tunnel: w503 -> [_ w511]
                    frame False {
                    }
                    frame True {
                      n141 = Divide(x=w513, y=w511) -> (x/y=w512:dbl)
                    }
                  }
                  n142 = Bundle By Name(cluster=w506, "Energy Cali.Energy Cali factor [mJ/Pixelsum]"=w504) -> (w507:T3)
                  n143 = call "PH_ImageCalibrator.set modified data.vi"("i ref in"=w509, "i attribute"=w507, "error in (no error)"=w508) -> ()  [unwired: 15 in, 2 out]
                }
                frame True {
                }
              }
            }
            frame #1 {
              n144 = while {
                tunnel: w518 -> [_]
                tunnel: [w526] -> w519
                tunnel: w520 -> [_]
                tunnel: w517 -> [w524]
                tunnel: [w524] -> w516
                tunnel: [w523] -> w515
                tunnel: w514 -> [w523]
                stop <- w525 continue-if-true
                # "do action"
                n145 = call "BaseSM.change state.vi"("default state"="Save result", "wait time [ms]"=0 ("wait time"), "i ref in"=w524) -> ("next state"=w526:string, "continue loop"=w525:bool)  [unwired: 13 in, 2 out]
              }
            }
            frame #2 {
              # "exit action"
            }
          }
        }
        frame "Save result" {
          n146 = stacked-sequence {
            tunnel: w533 -> [w545 w553 _]
            tunnel: [_ w552 _] -> w532
            tunnel: w531 -> [w537 w550 _]
            tunnel: [_ w549 _] -> w530
            tunnel: w529 -> [w546 w551 _]
            tunnel: w528 -> [w535 w547 _]
            tunnel: [_ w548 _] -> w527
            frame #0 {
              # "entry action"
              n147 = call "BaseSM.set state status.vi"("i ref in"=w537, "stateStatus"=w545, "ms timeout (10000)"=w546, "error in (no error)"=w535) -> ()  [unwired: 13 in, 3 out]
              n148 = call "PH_ImageCalibrator.get Text for Save Result Dialog.vi"("i ref in"=w537, "error in (no error)"=w535) -> ("i ref out"=w536:refnum<vi>, "User Dialog"=w539:string, "error out"=w534:errorcluster)  [unwired: 15 in]
              n149 = call "PH_ImageCalibrator.set User Dialog.vi"("i ref in"=w536, "State"=w545, "Text"=w539, "error in (no error)"=w534) -> ("i ref out"=w542:refnum<vi>, "error out"=w543:errorcluster)  [unwired: 14 in]
              n150 = call "BaseProcess.set pdc interval.vi"("i ref in"=w542, "PeriodicInterval [ms]"=-1 ("PeriodicInterval"), "error in (no error)"=w543) -> ("i ref out"=w541:refnum<vi>, "error out"=w540:errorcluster)  [unwired: 14 in, 1 out]
              n151 = call "PH_ImageCalibrator.set GUI elements.vi"("i ref in"=w541, "skip visible (true)"=FALSE, "error in (no error)"=w540) -> ()  [unwired: 15 in, 2 out]
            }
            frame #1 {
              n152 = while {
                tunnel: w551 -> [w554]
                tunnel: [w558] -> w552
                tunnel: w553 -> [_]
                tunnel: w550 -> [w556]
                tunnel: [w556] -> w549
                tunnel: [w555] -> w548
                tunnel: w547 -> [w555]
                stop <- w557 continue-if-true
                # "do action"
                n153 = call "BaseSM.change state.vi"("wait time [ms]"=w554, "i ref in"=w556) -> ("next state"=w558:string, "continue loop"=w557:bool)  [unwired: 14 in, 2 out]
              }
            }
            frame #2 {
              # "exit action"
            }
          }
        }
        frame Default {
          n154 = call "BaseSM.ProcState.vi"("i ref in"=w565, "state timeout [ms]"=w561, "state"=w560, "error in (no error)"=w563) -> ("i ref out"=w564:refnum<vi>, "next state"=w559:string, "error out"=w562:errorcluster)  [unwired: 13 in]
        }
      }
    }
    frame True {
      n155 = call "CoreLib.my to LV error.vi"("ErrorTypes"=CoreDefs.error_type."invalid reference") -> ("myErrorCluster"=w567:errorcluster)  [unwired: 17 in, 1 out]
    }
  }
  "i ref out" <- w8
  "next state" <- w6
  "error out" <- w3
